vi "Update comma separated field from string.vi"(6 "Field separator":string=",", 8 "error in (no error)":errorcluster, 9 "New field data":string, 10 "Field number (1-n)":u32, 11 "CSV string with field to update":string) -> (0 "error out":errorcluster, 3 "Updated csv string":string)   [LabVIEW 2013]
panel:
  out "After string":string
  out "before string":string
  out "Start of Nth field":i32
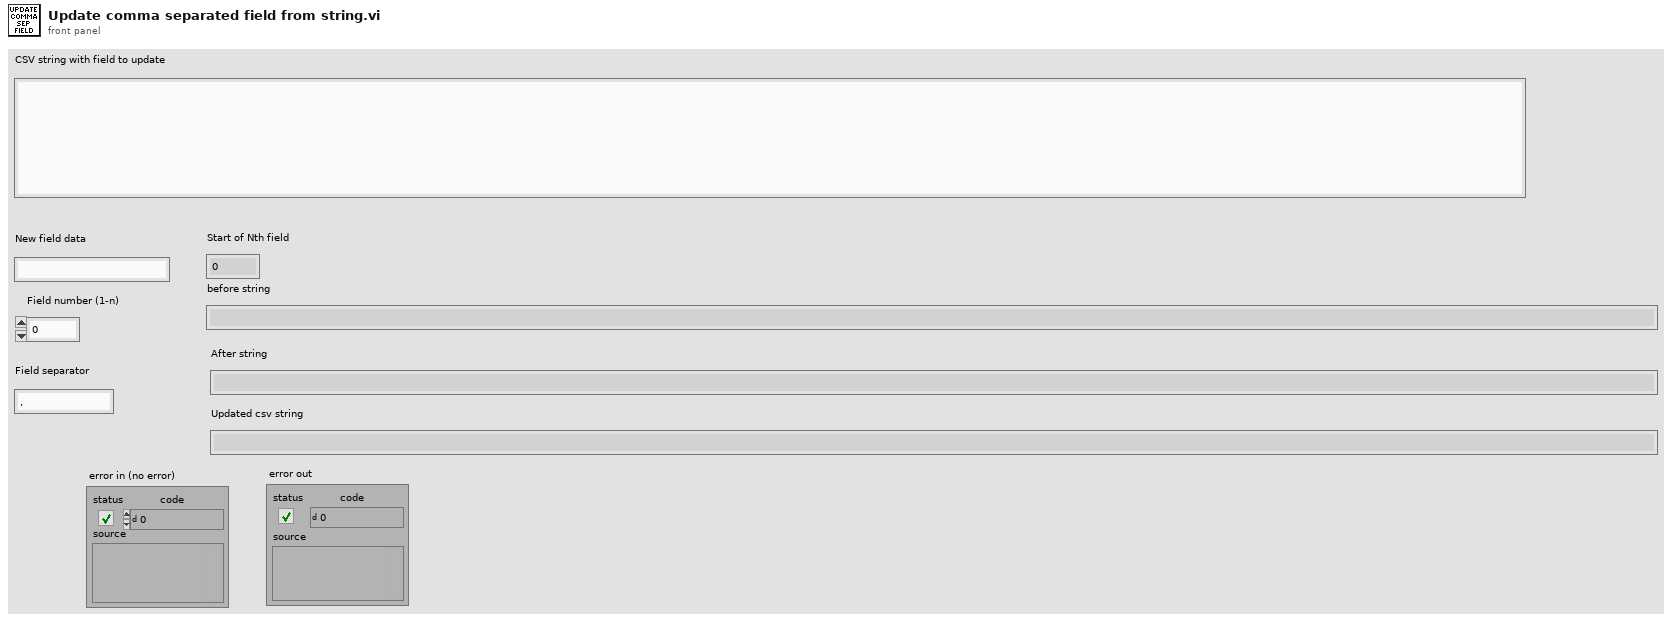
[diagram p1: front panel]
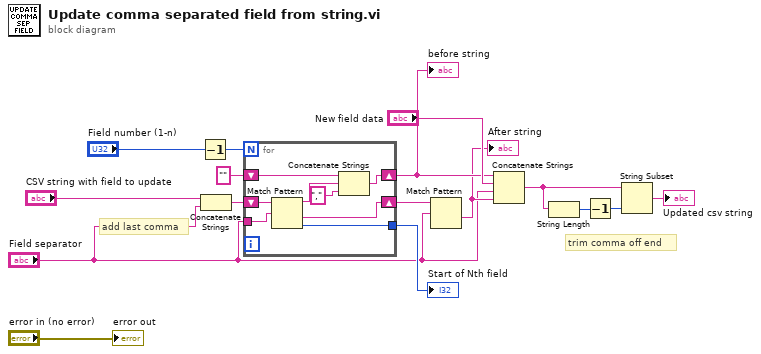
[diagram p0: block diagram]
diagram:
  # "trim comma off end"
  # "add last comma"
  n1 = Decrement(x="Field number (1-n)") -> (x-1=w10:u32)
  n2 = Concatenate Strings("CSV string with field to update", "Field separator") -> (w16:string)
  n3 = for {
    N: w10 -> [_]
    shift-right: [w21] -> w7
    shift-left: w16 -> [w24]
    tunnel: "Field separator" -> [w23]
    tunnel: [w22] -> w13
    shift-right: [w18] -> w8
    shift-left: "" -> [w20]
    n4 = Match Pattern(string=w24, regular expression=w23) -> (before substring=w19:string, after substring=w21:string, offset past match=w22:i32)  [unwired: 1 in, 1 out]
    n5 = Concatenate Strings(w20, w19, "," ("string")) -> (w18:string)
  }
  "Start of Nth field" <- w13
  "before string" <- w8
  n6 = Match Pattern(string=w7, regular expression="Field separator") -> (after substring=w6:string)  [unwired: 1 in, 3 out]
  "After string" <- w6
  n7 = Concatenate Strings(w8, "New field data", "Field separator", w6) -> (w2:string)
  n8 = String Length(string=w2) -> (length=w4:i32)
  n9 = Decrement(x=w4) -> (x-1=w3:i32)
  n10 = String Subset(string=w2, length (rest)=w3) -> (substring=→"Updated csv string":string)  [unwired: 1 in]
  "error out" <- "error in (no error)"
